vi "Recurse Wins.vi"(10 "Pile":refnum<class "Card.lvclass">[](array[class]), 11 "Card in":refnum<class "Card.lvclass">) -> (3 "New Cards":refnum<class "Card.lvclass">[](array[class]))   [LabVIEW 2020]
uses:
  Card.lvclass
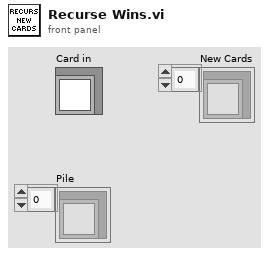
[diagram p1: front panel]
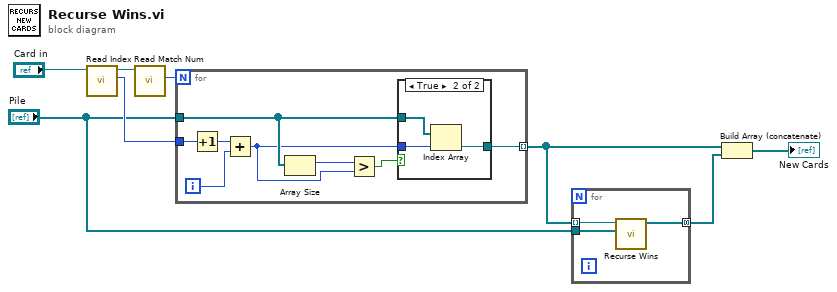
[diagram p0: block diagram]
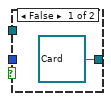
[diagram p2: hidden frame]
diagram:
  n1 = call-dynamic "Read Index.vi"("Card in"="Card in") -> ("Index"=w8:i32, "Card out"=w7:refnum<class "Card.lvclass">)  [unwired: 8 in, 1 out]
  n2 = call-dynamic "Read Match Num.vi"("Card in"=w7) -> ("Matches"=w5:i32)  [unwired: 8 in, 2 out]
  n3 = for {
    N: w5 -> [_]
    tunnel: "Pile" -> [w12]
    tunnel: [w14] -> w3 mode=indexing
    tunnel: w8 -> [w13]
    i -> [w15]
    n4 = Increment(x=w13) -> (x+1=w16:i32)
    n5 = Add(x=w16, y=w15) -> (x+y=w10:i32)
    n6 = Array Size(array=w12) -> (size(s)=w11:i32)
    n7 = Greater?(x=w11, y=w10) -> (0:w9:bool)
    n8 = case shown="True" w9 {
      tunnel: [refnum<class "Card.lvclass"> refnum ("Card") w20] -> w14
      tunnel: w12 -> [_ w19]
      tunnel: w10 -> [_ w18]
      frame False {
      }
      frame True {
        n9 = Index Array(array=w19, index=w18) -> (element=w20:refnum<class "Card.lvclass">)
      }
    }
  }
  n10 = for {
    tunnel: "Pile" -> [w23]
    tunnel: w3 -> [w22] mode=indexing
    tunnel: [w21] -> w2 mode=concatenating
    n11 = call "Recurse Wins.vi"("Pile"=w23, "Card in"=w22) -> ("New Cards"=w21:refnum<class "Card.lvclass">[])  [unwired: 9 in]
  }
  n12 = Build Array (concatenate)(w3, w2) -> (→"New Cards":refnum<class "Card.lvclass">[])
